vi "Foot conversion.vi"(1 "Feet":dbl format="%#_13g") -> (0 "Tach Counts":dbl)   [LabVIEW 2014]
uses:
  Global Constants.vi
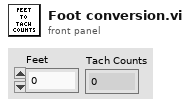
[diagram p1: front panel]
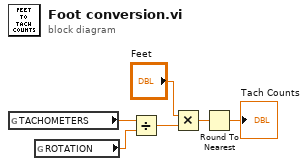
[diagram p0: block diagram]
diagram:
  n1 = global read "Global Constants.vi" "TACHOMETERS"() -> (w2:dbl)
  n2 = global read "Global Constants.vi" "ROTATION"() -> (w1:dbl)
  n3 = Divide(x=w2, y=w1) -> (x/y=w6:dbl)
  n4 = Multiply(x="Feet", y=w6) -> (x*y=w4:dbl)
  n5 = Round To Nearest(number=w4) -> (nearest integer value=→"Tach Counts":dbl)
